vi "Update Step Action Visibility.vi"(8 "Actions visible":bool, 9 "Step tag":string, 10 "TreeControl in":refnum<vi>, 11 "Step Settings":T1) -> ()   [LabVIEW 2020, in "Output Sequencer.lvlib" / "Settings UI.lvclass"]
uses:
  Settings UI.lvclass
  Types/Step Settings.ctl
  Types/Tree Index Enum.ctl
  Globals/Global Tree Data.vi
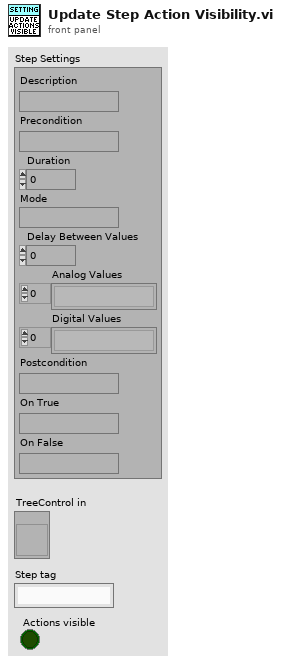
[diagram p1: front panel]
types:
  T1 = typedef "Output Sequencer.lvlib/Settings UI.lvclass/Step Settings.ctl" = cluster{"Description":string, "Precondition":string, "Duration":dbl, "Mode":string, "Delay Between Values":dbl, "Analog Values":string[], "Digital Values":string[], "Postcondition":string, "On True":string, "On False":string}
  T2 = typedef "Output Sequencer.lvlib/Settings UI.lvclass/Tree Index Enum.ctl" = enum16{"General Settings", "Num Steps", "Num Analog", "Num Digital", "Show Confirmation", "Interp Priority", "Adv Timing", "Enable Conditions", "Seq Execution", "Reset Test Start", "Only When Test", "Delay After Test", "Start condition", "Re-triggering", "Stop condition", "Stop After Cycles", "Stop Values", "Default Values", "Default Analog", "Default Digital", "Steps", "Step #", "Description", "Precondition", "Duration", "Mode", "Delay Between Vals", "Analog Values", "Digital Values", "Postcondition", "On True", "On False"}
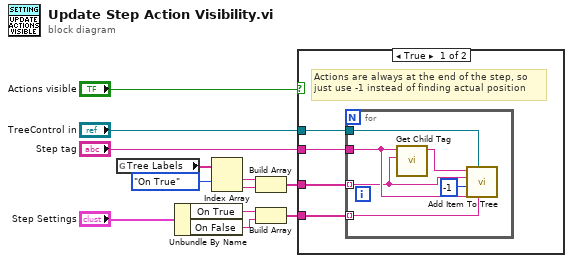
[diagram p0: block diagram]
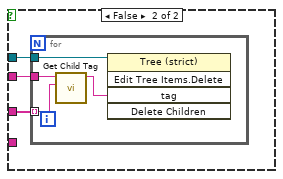
[diagram p2: hidden frame]
diagram:
  n1 = global read "Global Tree Data.vi" "Tree Labels"() -> (w10:string[])
  n2 = Unbundle By Name("Step Settings") -> ("On True"=w3:string, "On False"=w4:string)
  n3 = Index Array(array=w10, index #1=Tree_Index_Enum."On True" ("Tree Index Enum")) -> (element #1=w9:string, element #2=w8:string)  [unwired: 1 in]
  n4 = Build Array(w9, w8) -> (w12:string[])
  n5 = Build Array(w3, w4) -> (w2:string[])
  n6 = case shown="True" "Actions visible" {
    tunnel: "TreeControl in" -> [w14 w25]
    tunnel: w12 -> [w16 w24]
    tunnel: "Step tag" -> [w15 w23]
    tunnel: w2 -> [w13 _]
    frame True {
      # "Actions are always at the end of the step, so\njust use -1 instead of finding actual position"
      n7 = for {
        tunnel: w16 -> [w18] mode=indexing
        tunnel: w13 -> [w21] mode=indexing
        tunnel: w15 -> [w19]
        tunnel: w14 -> [w22]
        n8 = call "Get Child Tag.vi"("Child label"=w18, "Parent tag"=w19) -> ("Child tag"=w17:string)  [unwired: 9 in]
        n9 = call "Add Item To Tree.vi"("Child Text"=w21, "TreeControl in"=w22, "Parent Tag"=w19, "Child Position"=-1, "Left Cell String"=w18, "Child Tag in"=w17) -> ()  [unwired: 5 in, 1 out]
      }
    }
    frame False {
      n10 = for {
        tunnel: w25 -> [w29]
        tunnel: w24 -> [w28] mode=indexing
        tunnel: w23 -> [w27]
        n11 = call "Get Child Tag.vi"("Child label"=w28, "Parent tag"=w27) -> ("Child tag"=w26:string)  [unwired: 9 in]
        n12 = invoke class="Tree (strict)" method="Edit Tree Items.Delete"(reference=w29, "tag"=w26) -> ()  [unwired: 3 in, 5 out]
      }
    }
  }
